vi "Read Channels.vi"(8 "error in":errorcluster, 11 "module in":refnum<class "Module.lvclass">) -> (0 "error out":errorcluster, 2 "channels":refnum<class "Channel.lvclass">[](array[class]), 3 "module out":refnum<class "Module.lvclass">)   [LabVIEW 2017, in "Scan Engine Scripting.lvlib" / "Module.lvclass"]
doc: "Reads the channels from the private data of the module."
uses:
  Module.lvclass
  Channel Classes/Channel/Channel.lvclass
  Module.lvclass/Module.ctl
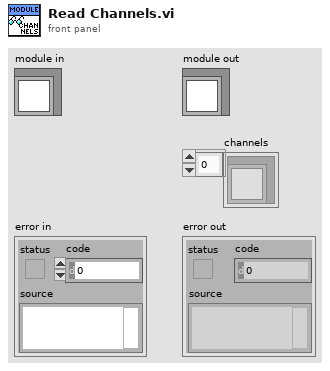
[diagram p1: front panel]
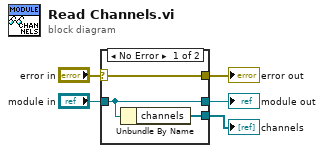
[diagram p0: block diagram]
diagram:
  n1 = case shown="No Error" "error in" {
    selector: "error in" -> [w8 w9]
    tunnel: [w8 w9] -> w4
    tunnel: [w7 w10] -> w2
    tunnel: "module in" -> [w7 w10]
    tunnel: [w6 _] -> w1
    frame No Error {
      n2 = Unbundle By Name(w7) -> ("channels"=w6:refnum<class "Channel.lvclass">[])
    }
    frame Error {
    }
  }
  "error out" <- w4
  "module out" <- w2
  "channels" <- w1
